vi "Fine rampa sinus penta.vi"() -> ()   [LabVIEW 2019]
panel:
  out "DISABILITA STOP FRENO":bool
  out "BANCO 300KW":bool
  out "LIMITAZIONE AFE":bool
  out "Fine Rampa DCREG":bool
  out "Fine Rampa sinus penta":bool
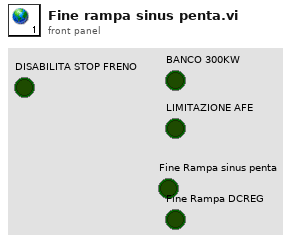
[diagram p1: front panel]
diagram:
